vi "GUI_EPS Interface.vi"() -> ()   [LabVIEW 2013]
uses:
  Shared/GUI_Template/GUI_master/tcp_new_data_event.ctl
  Shared/GUI_Template/GUI_master/tcp new data cluster.ctl
panel:
  out "tcp data event":T1
  in  "Refresh Button":bool
  out "statusfloatarrayname.var 1-0::1":string caption="NAME"
  out "statusfloatarrayname.var 1-1::1":string caption="NAME"
  out "statusfloatarray.var 1-0::1":dbl caption="Value" min=0.0 max=0.0
  out "statusfloatarray.var 1-1::1":dbl caption="Value" min=0.0 max=0.0
  out "statusintegerarray.var 1-1::1":i32 caption="Value" min=0 max=0
  out "statusintegerarray.var 1-0::1":i32 caption="Value" min=0 max=10000
  out "statusintegerarrayname.var 1-0::1":string caption="NAME"
  out "statusintegerarrayname.var 1-1::1":string caption="NAME"
  out "statusboolarrayname1.var 1-1::1":string caption="NAME"
  out "statusboolarrayname1.var 1-0::1":string caption="NAME"
  out "statusboolarray1.var 1-1::1":enum16{"off", "on"}(ring) caption="Value"
  out "statusboolarray1.var 1-0::1":enum16{"off", "on"}(ring) caption="Value"
  out "name.var 1-0::1":string caption="NAME"
  in  "variable.var 1-0::1":enum16{"off", "on"}(ring) caption="Toggle"
  in  "insert tag":bool=TRUE
  in  "stop":bool
  in  "GUIdevice 1":string="71146 EPS Interface"
  # "BOOL1"
  # "INTEGER"
  # "FLOAT"
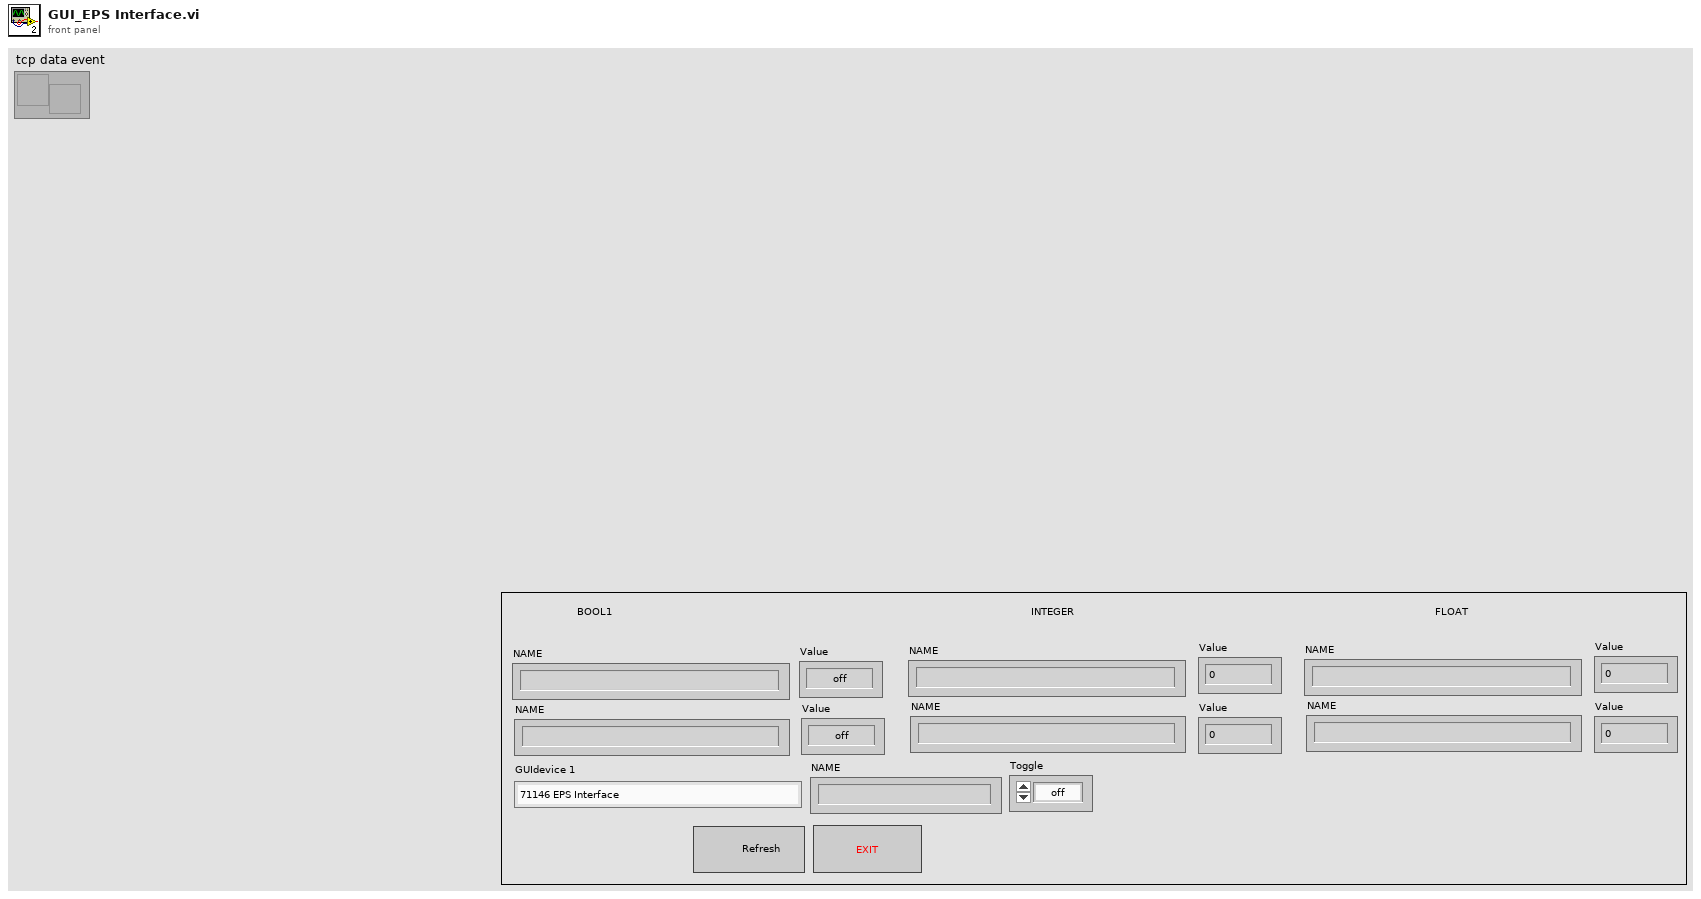
[diagram p1: front panel]
types:
  T1 = typedef "tcp_new_data_event.ctl" = refnum<user-event>
  T2 = enum32{"invalid app kind", "Development System", "Run Time System", "Student Edition", "Embedded LabVIEW", "Evaluation", "Custom"}
  T3 = typedef "tcp new data cluster.ctl" = cluster{"EventEnum":enum16{"new data", "connection status update"}, "Device name":string}
  T4 = enum32{"Invalid", "Standard", "Closed", "Hidden", "Minimized", "Maximized"}
  T5 = cluster{"Core":cluster{"Current VI Reference":refnum<vi>, "Close Panel on Exit?":bool}, "Your Boolean data":bool, "Your string data":string, "SuperGUI":cluster{"STOP queue":refnum<queue>, "SuperGUI ref":refnum<vi>}}
  T6 = cluster{"STOP queue":refnum<queue>, "SuperGUI ref":refnum<vi>}
  T7 = cluster{"Current VI Reference":refnum<vi>, "Close Panel on Exit?":bool}
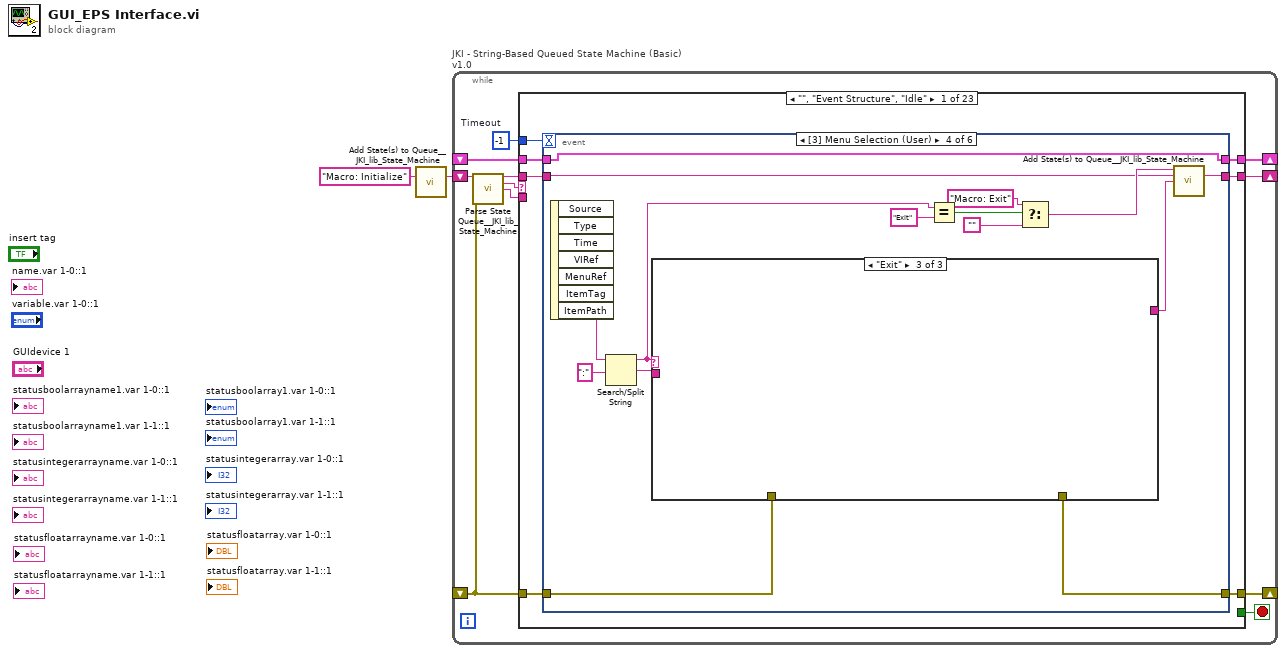
[diagram p0: block diagram]
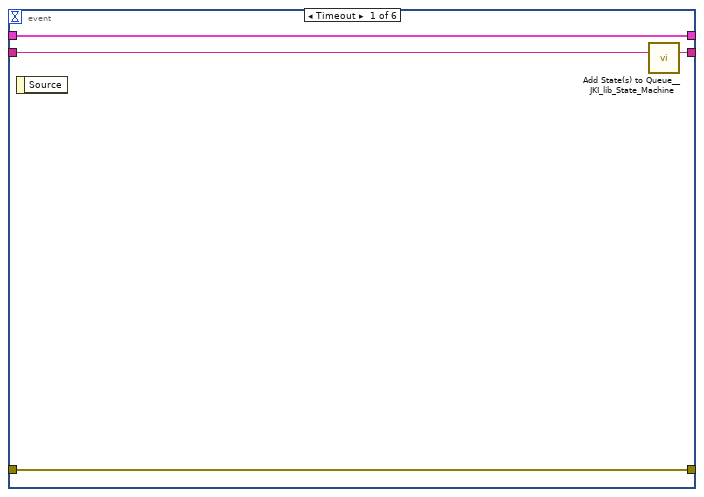
[diagram p2: hidden frame]
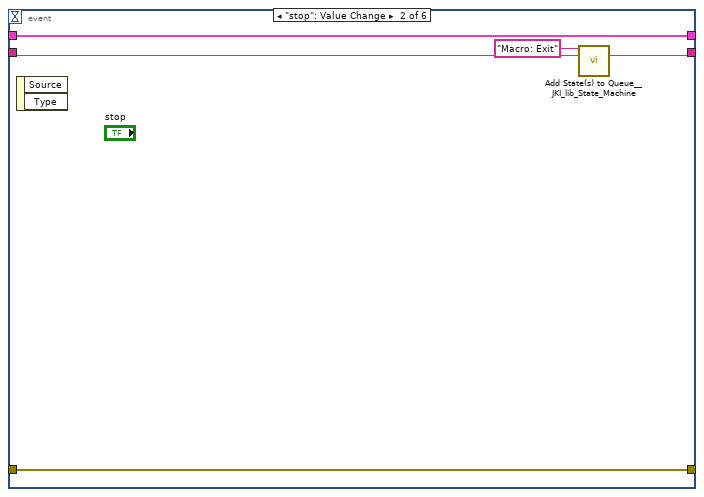
[diagram p3: hidden frame]
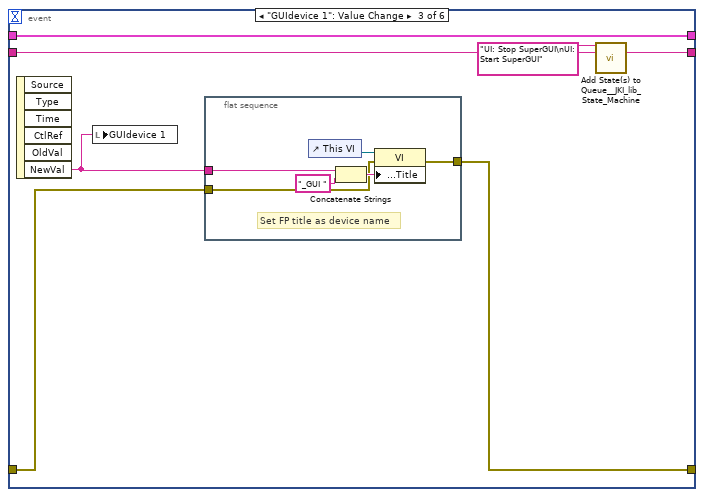
[diagram p4: hidden frame]
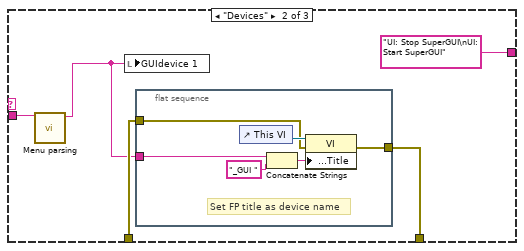
[diagram p6: hidden frame]
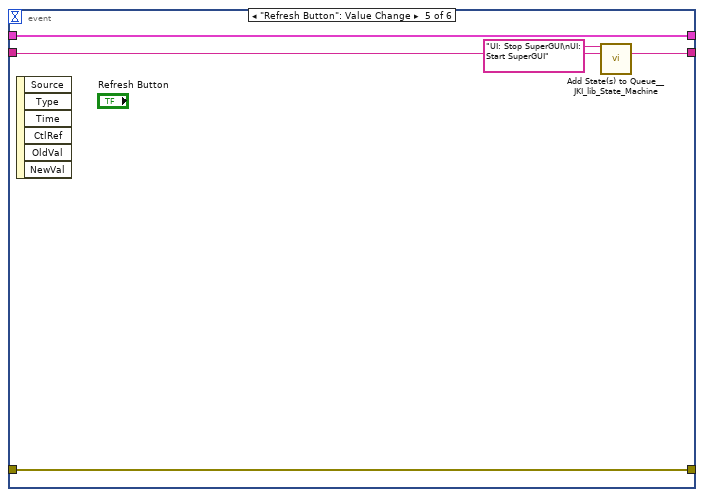
[diagram p7: hidden frame]
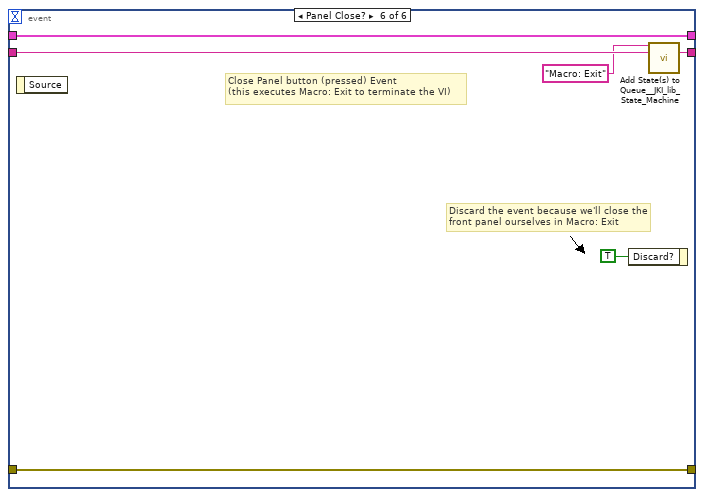
[diagram p8: hidden frame]
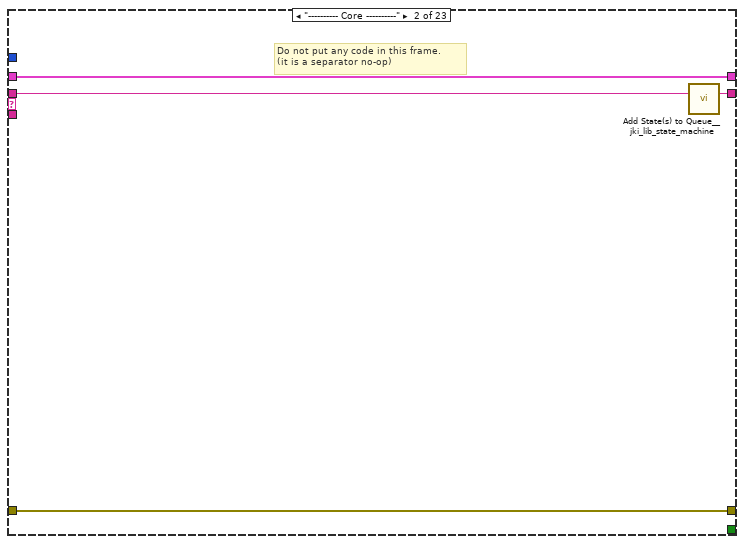
[diagram p9: hidden frame]
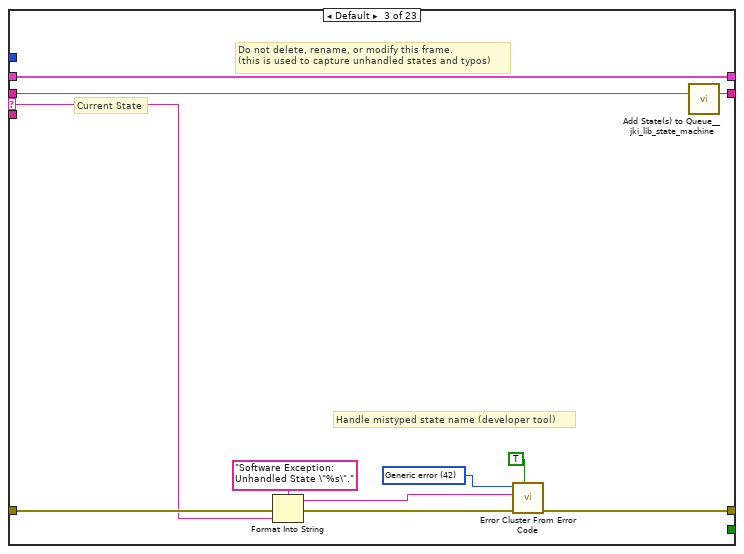
[diagram p10: hidden frame]
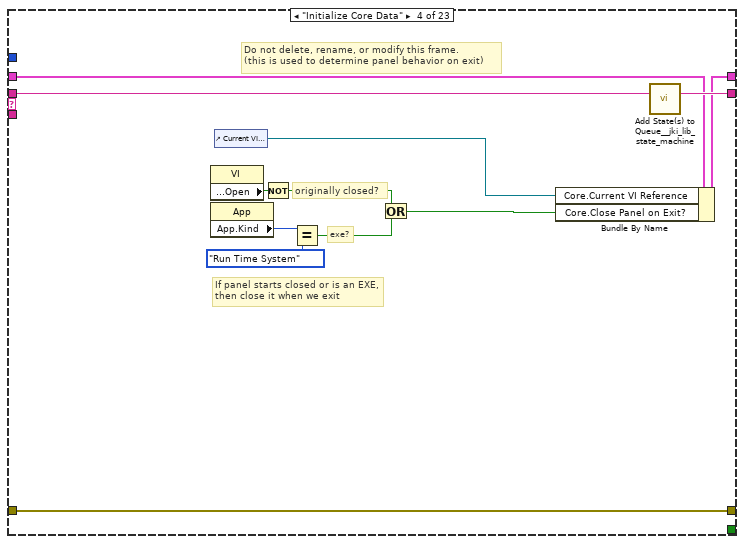
[diagram p11: hidden frame]
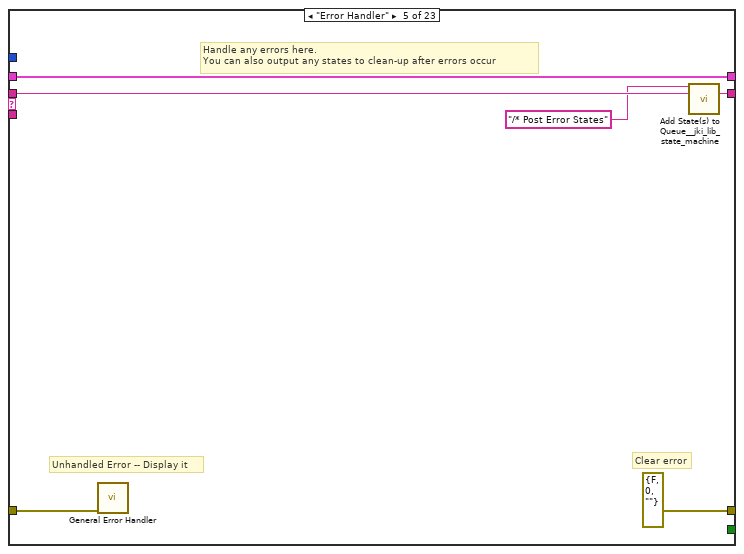
[diagram p12: hidden frame]
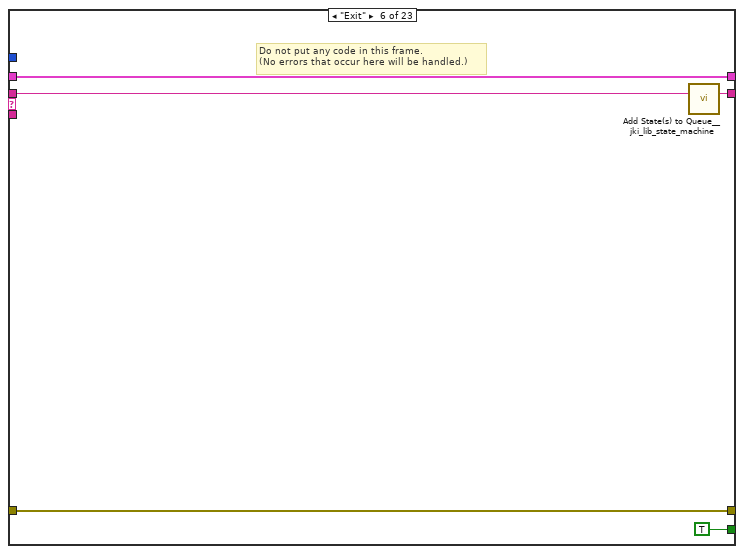
[diagram p13: hidden frame]
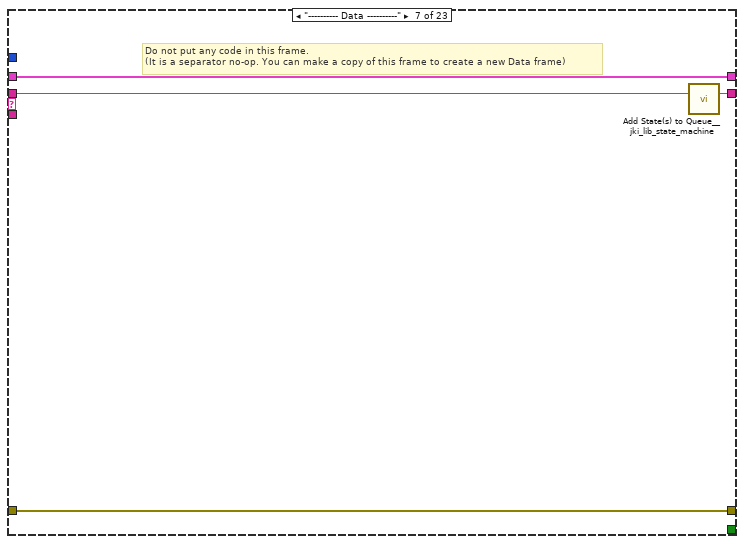
[diagram p14: hidden frame]
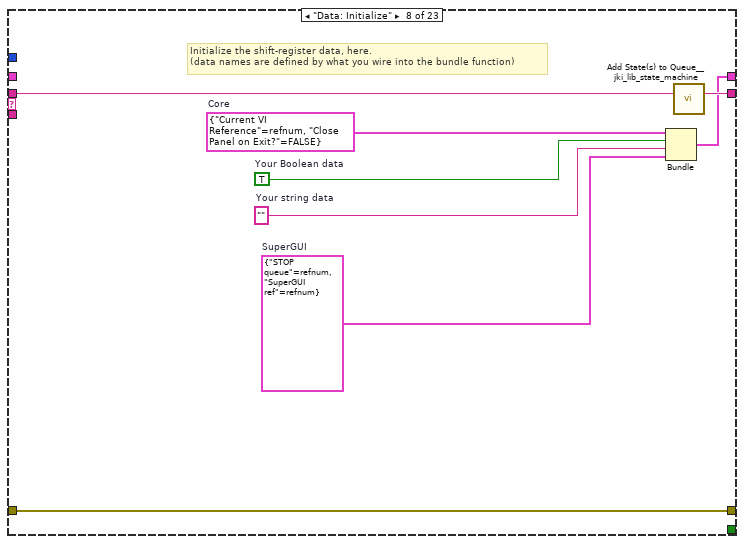
[diagram p15: hidden frame]
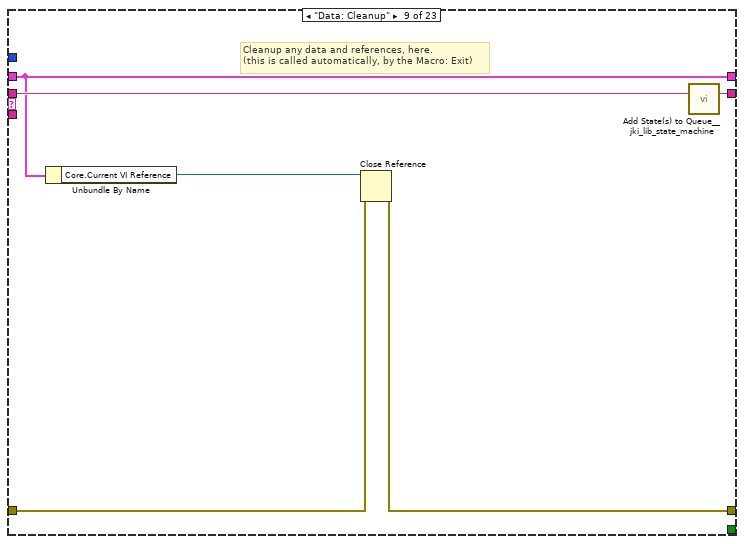
[diagram p16: hidden frame]
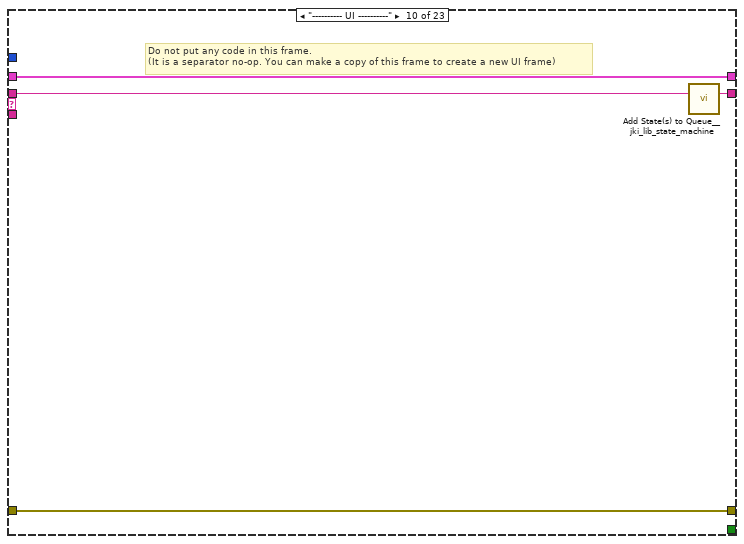
[diagram p17: hidden frame]
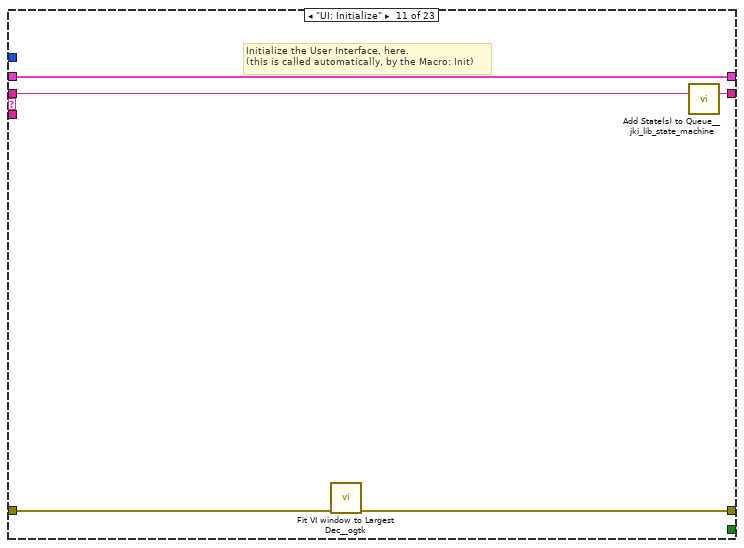
[diagram p18: hidden frame]
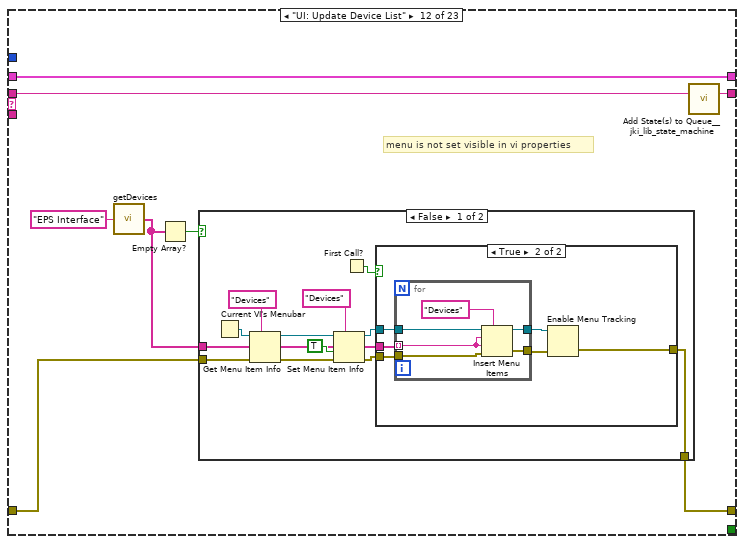
[diagram p19: hidden frame]
diagram:
  n1 = call <vilib>:"Add State(s) to Queue__JKI_lib_State_Machine.vi"("State(s) in (\"\")"="Macro: Initialize") -> ("States Out"=w2:string)  [unwired: 14 in]
  n2 = while "JKI - String-Based Queued State Machine (Basic) v1.0" {
    shift-right: [w6] -> _
    shift-left: _ -> [w5]
    shift-right: [w9] -> _
    shift-left: _ -> [w3]
    shift-right: [w8] -> _
    shift-left: w2 -> [w10]
    stop <- w7 stop-if-true
    w4 = -1  # Timeout
    n3 = call <vilib>:"Parse State Queue__JKI_lib_State_Machine.vi"("State Queue"=w10, "Error In (no error)"=w3) -> ("Remaining States"=w12:string, "Current State"=w13:string, "Arguments"=w11:string)  [unwired: 11 in]
    n4 = case shown="\"\", \"Event Structure\", \"Idle\"" w13 {
      selector: w13 -> [_ _ w86 _ _ _ _ _ _ _ _ _ _ _ _ _ _ _ _ _ _ _ _]
      tunnel: w12 -> [w20 w85 w90 w108 w114 w119 w123 w131 w137 w141 w146 w154 w186 w220 w228 w234 w245 w271 w276 w286 w290 w294 w298]
      tunnel: w11 -> [_ _ _ _ _ _ _ _ _ _ _ _ _ _ _ w229 w239 _ _ _ _ _ _]
      tunnel: w5 -> [w18 w82 w88 w99 w111 w117 w120 _ w132 w138 w144 w152 w184 w211 w223 w232 w241 w268 w273 w283 w287 w291 w295]
      tunnel: [w17 w83 w92 w105 errorcluster {"status"=FALSE, "code"=0, "source"=""} ("error out") w116 w121 w128 w133 w139 w142 w150 w181 w204 w221 w230 w242 w269 w274 w284 w288 w292 w296] -> w9
      tunnel: w3 -> [w16 w83 w91 w105 w110 w116 w121 w128 w134 w139 w143 w151 w182 w205 w222 w231 w243 w269 w274 w284 w288 w292 w296]
      tunnel: [w19 w84 w89 w107 w113 w118 w122 w130 w136 w140 w145 w153 w185 w219 w227 w233 w244 w270 w275 w285 w289 w293 w297] -> w8
      tunnel: [_ _ _ _ _ TRUE _ _ _ _ _ _ _ _ _ _ _ _ _ _ _ _ _] -> w7
      tunnel: [w15 w82 w88 w106 w111 w117 w120 w129 w132 w138 w144 w152 w184 w210 w223 w232 w241 w268 w273 w283 w287 w291 w295] -> w6
      tunnel: w4 -> [w14 _ _ _ _ _ _ _ _ _ _ _ _ _ _ _ _ _ _ _ _ _ _]
      frame "", "Event Structure", "Idle" {
        n5 = event shown="[3] Menu Selection (User)" {
          selector: _ -> [_ _ _ _ _ _]
          dyn-events: _ -> [_ _ _ _ _ _]
          timeout: w14 -> [_ _ _ _ _ _]
          tunnel: w20 -> [w24 w27 w33 w51 w73 w81]
          tunnel: [w23 w26 w32 w50 w72 w80] -> w19
          tunnel: w18 -> [w21 w29 w36 w57 w75 w78]
          tunnel: [w22 w28 w34 w44 w74 w79] -> w17
          tunnel: w16 -> [w22 w28 w35 w45 w74 w79]
          tunnel: [w21 w29 w36 w57 w75 w78] -> w15
          event Timeout {
            n6 = event-data() -> ()  [unwired: 1 in, 1 out]
            n7 = call <vilib>:"Add State(s) to Queue__JKI_lib_State_Machine.vi"("State(s) in (\"\")"=w24) -> ("States Out"=w23:string)  [unwired: 14 in]
          }
          event "stop": Value Change {
            n8 = event-data() -> ()  [unwired: 1 in, 2 out]
            n9 = call <vilib>:"Add State(s) to Queue__JKI_lib_State_Machine.vi"("State(s) in Front (\"\")"="Macro: Exit", "State(s) in (\"\")"=w27) -> ("States Out"=w26:string)  [unwired: 13 in]
          }
          event "GUIdevice 1": Value Change {
            n10 = event-data() -> ("NewVal"=w30:string)  [unwired: 1 in, 5 out]
            n11 = local write "GUIdevice 1"(w30) -> ()
            n12 = flat-sequence {
              tunnel: [w39] -> w34
              tunnel: w35 -> [w38]
              tunnel: w30 -> [w37]
              frame #0 {
                # "Set FP title as device name"
                n13 = control-ref of="This VI"() -> (w42:refnum<vi>)
                n14 = Concatenate Strings(w37, "_GUI ") -> (w41:string)
                n15 = property class="VI"(reference=w42, error in=w38, "Front Panel.Title"=w41) -> (error out=w39:errorcluster)  [unwired: 1 out]
              }
            }
            n16 = call <vilib>:"Add State(s) to Queue__JKI_lib_State_Machine.vi"("State(s) in Front (\"\")"="UI: Stop SuperGUI\nUI: Start SuperGUI", "State(s) in (\"\")"=w33) -> ("States Out"=w32:string)  [unwired: 13 in]
          }
          event Menu Selection (User) {
            n17 = event-data() -> ("ItemPath"=w47:string)  [unwired: 1 in, 6 out]
            n18 = Search/Split String(string=w47, search string/char (-)=":") -> (substring before match=w43:string, match + rest of string=w46:string)  [unwired: 1 in, 1 out]
            n19 = case shown="\"Exit\"" w43 {
              tunnel: w46 -> [_ w63 _]
              tunnel: w45 -> [w58 w62 w70]
              tunnel: [w58 w61 w70] -> w44
              tunnel: [_ "UI: Stop SuperGUI\nUI: Start SuperGUI" _] -> w49
              frame "", Default {
              }
              frame "Devices" {
                n20 = call "Menu parsing.vi"("ItemPath"=w63) -> ("ItemPath"=w59:string)  [unwired: 9 in, 1 out]
                n21 = local write "GUIdevice 1"(w59) -> ()
                n22 = flat-sequence {
                  tunnel: [w66] -> w61
                  tunnel: w62 -> [w65]
                  tunnel: w59 -> [w64]
                  frame #0 {
                    # "Set FP title as device name"
                    n23 = control-ref of="This VI"() -> (w69:refnum<vi>)
                    n24 = Concatenate Strings(w64, "_GUI ") -> (w68:string)
                    n25 = property class="VI"(reference=w69, error in=w65, "Front Panel.Title"=w68) -> (error out=w66:errorcluster)  [unwired: 1 out]
                  }
                }
              }
              frame "Exit" {
              }
            }
            n26 = Equal?(x=w43, y="Exit") -> (x = y?=w55:bool)
            n27 = Select(t="Macro: Exit", s=w55, f="") -> (s? t:f=w52:string)
            n28 = call <vilib>:"Add State(s) to Queue__JKI_lib_State_Machine.vi"("State(s) in Front (\"\")"=w52, "State(s) in (\"\")"=w51, "State(s) at Back (\"\")"=w49) -> ("States Out"=w50:string)  [unwired: 12 in]
          }
          event "Refresh Button": Value Change {
            n29 = event-data() -> ()  [unwired: 1 in, 6 out]
            n30 = call <vilib>:"Add State(s) to Queue__JKI_lib_State_Machine.vi"("State(s) in Front (\"\")"="UI: Stop SuperGUI\nUI: Start SuperGUI", "State(s) in (\"\")"=w73) -> ("States Out"=w72:string)  [unwired: 13 in]
          }
          event Panel Close? {
            # "Discard the event because we'll close the front panel ourselves in Macro: Exit"
            # "Close Panel button (pressed) Event\n(this executes Macro: Exit to terminate the VI)"
            n31 = event-data() -> ()  [unwired: 1 in, 1 out]
            n32 = event-data("Discard?"=TRUE) -> ()  [unwired: 1 in, 1 out]
            n33 = call <vilib>:"Add State(s) to Queue__JKI_lib_State_Machine.vi"("State(s) in Front (\"\")"="Macro: Exit", "State(s) in (\"\")"=w81) -> ("States Out"=w80:string)  [unwired: 13 in]
          }
        }
      }
      frame "---------- Core ----------" {
        # "Do not put any code in this frame.\n(it is a separator no-op)"
        n34 = call <vilib>:"Add State(s) to Queue__jki_lib_state_machine.vi"("State(s) in (\"\")"=w85) -> ("States Out"=w84:string)  [unwired: 14 in]
      }
      frame Default {
        w95 = 42 items=["No error", "Argument error", "Memory is full", "Out of zone", "End of file", "File already open", "Generic file I/O error", "File not found", "File permission error", "Disk is full", "Duplicate path", "Too many files open", "System feature not enabled", "Resource file not found", "Cannot add resource", "Resource not found", "Image not found", "Image memory error", "Pen does not exist", "Config type invalid", "Config token not found", "Config parse error", "Config memory error", "Bad external code format", "Bad external code offset", "External code not present", "Null window", "Destroy window error", "Null menu", "Print aborted", "Bad print record", "Print driver error", "Windows error during printing", "Memory error during printing", "Print dialog error", "Generic print error", "Invalid device refnum", "Device not found", "Device parameter error", "Device unit error", "Cannot open device", "Device call aborted", "Generic error", "Cancelled by user", "Object ID too low", "Object ID too high", "Object not in heap", "Unknown heap", "Unknown object (invalid DefProc)", "Unknown object (DefProc not in table)", "Message out of range", "Invalid (null) method", "Unknown message", "Manager call not supported", "Bad address", "Network operation in progress", "Network operation timed out", "Connection is busy", "Network attribute not supported", "Network error", "Address in use", "System out of memory", "Connection aborted", "Connection refused", "Not connected", "Already connected", "Connection closed", "Initialization error (interapplication manager)", "Bad occurrence", "Wait on unbound occurrence handler", "Occurrence queue overflow", "Datalog type conflict", "Unused", "Unrecognized type (interapplication manager)", "Memory corrupt", "Failed to make temporary DLL", "Old CIN version", "Drag socket not found", "Failed to load drop-object", "Failed to register OLE object", "Failed to release OLE object", "Format specifier type mismatch", "Unknown format specifier", "Too few format specifiers", "Too many format specifiers", "Scan failed", "Newer CIN version", "Error converting to variant", "Runtime menu error", "Password tampered", "Variant attribute not found", "Incompatible variant data type", "Event data is not available", "Event Store is not present", "Occurrence is not found", "Event Queue is not created", "Event info is not available", "Refnum passed is NULL", "Error retrieving Class GUID", "Error retrieving CoClass GUID", "Error retrieving TypeLib GUID.", "Bad built application magic bytes.", "Specific driver is different from the specific driver associated with the Logical Name.", "There is no session opened to the class driver.", "Max Error", "MAX - Error with config objects", "MAX - Error loading configuration", "MAX - Group not supported"]
        # "Current State"
        # "Do not delete, rename, or modify this frame.\n(this is used to capture unhandled states and typos)"
        # "Handle mistyped state name (developer tool)"
        n35 = Format Into String(format string="Software Exception: Unhandled State \"%s\"." ("message"), error in=w91, w86) -> (resulting string=w94:string, error out=w93:errorcluster)  [unwired: 1 in]
        n36 = call <vilib>:"Error Cluster From Error Code.vi"("show call chain? (False)"=TRUE, "error in (no error)"=w93, "error message (\"\")"=w94, "error code (0)"=w95) -> ("error out"=w92:errorcluster)  [unwired: 5 in]
        n37 = call <vilib>:"Add State(s) to Queue__jki_lib_state_machine.vi"("State(s) in (\"\")"=w90) -> ("States Out"=w89:string)  [unwired: 14 in]
      }
      frame "Initialize Core Data" {
        # "Do not delete, rename, or modify this frame.\n(this is used to determine panel behavior on exit)"
        # "originally closed?"
        # "exe?"
        # "If panel starts closed or is an EXE, then close it when we exit"
        n38 = property class="VI"() -> ("Front Panel.Open"=w104:bool)  [unwired: 2 in, 2 out]
        n39 = property class="App"() -> ("App.Kind"=w103:T2)  [unwired: 2 in, 2 out]
        n40 = control-ref of="Current VI Reference"() -> (w97:refnum<vi>)
        n41 = Not(x=w104) -> (.not. x?=w101:bool)
        n42 = Equal?(x=w103, y=T2."Run Time System" ("Application:Kind")) -> (x = y?=w100:bool)
        n43 = Or(x=w101, y=w100) -> (x .or. y?=w98:bool)
        n44 = Bundle By Name(cluster=w99, "Core.Current VI Reference"=w97, "Core.Close Panel on Exit?"=w98) -> (w106:T5)
        n45 = call <vilib>:"Add State(s) to Queue__jki_lib_state_machine.vi"("State(s) in (\"\")"=w108) -> ("States Out"=w107:string)  [unwired: 14 in]
      }
      frame "Error Handler" {
        # "Unhandled Error -- Display it"
        # "Handle any errors here.\nYou can also output any states to clean-up after errors occur"
        # "Clear error"
        n46 = call <vilib>:"General Error Handler.vi"("error in (no error)"=w110) -> ()  [unwired: 10 in, 5 out]
        n47 = call <vilib>:"Add State(s) to Queue__jki_lib_state_machine.vi"("State(s) in Front (\"\")"="/* Post Error States", "State(s) in (\"\")"=w114) -> ("States Out"=w113:string)  [unwired: 13 in]
      }
      frame "Exit" {
        # "Do not put any code in this frame.\n(No errors that occur here will be handled.)"
        n48 = call <vilib>:"Add State(s) to Queue__jki_lib_state_machine.vi"("State(s) in (\"\")"=w119) -> ("States Out"=w118:string)  [unwired: 14 in]
      }
      frame "---------- Data ----------" {
        # "Do not put any code in this frame.\n(It is a separator no-op. You can make a copy of this frame to create a new Data frame)"
        n49 = call <vilib>:"Add State(s) to Queue__jki_lib_state_machine.vi"("State(s) in (\"\")"=w123) -> ("States Out"=w122:string)  [unwired: 14 in]
      }
      frame "Data: Initialize" {
        w124 = T6 {"STOP queue"=refnum, "SuperGUI ref"=refnum}  # SuperGUI
        w125 = T7 {"Current VI Reference"=refnum, "Close Panel on Exit?"=FALSE}  # Core
        w127 = TRUE  # Your Boolean data
        w126 = ""  # Your string data
        # "Initialize the shift-register data, here.\n(data names are defined by what you wire into the bundle function)"
        n50 = Bundle("Core"=w125, "Your Boolean data"=w127, "Your string data"=w126, "SuperGUI"=w124) -> (w129:T5)  [unwired: 1 in]
        n51 = call <vilib>:"Add State(s) to Queue__jki_lib_state_machine.vi"("State(s) in (\"\")"=w131) -> ("States Out"=w130:string)  [unwired: 14 in]
      }
      frame "Data: Cleanup" {
        # "Cleanup any data and references, here.\n(this is called automatically, by the Macro: Exit)"
        n52 = Unbundle By Name(w132) -> ("Core.Current VI Reference"=w135:refnum<vi>)
        n53 = Close Reference(reference=w135, error in (no error)=w134) -> (error out=w133:errorcluster)
        n54 = call <vilib>:"Add State(s) to Queue__jki_lib_state_machine.vi"("State(s) in (\"\")"=w137) -> ("States Out"=w136:string)  [unwired: 14 in]
      }
      frame "---------- UI ----------" {
        # "Do not put any code in this frame.\n(It is a separator no-op. You can make a copy of this frame to create a new UI frame)"
        n55 = call <vilib>:"Add State(s) to Queue__jki_lib_state_machine.vi"("State(s) in (\"\")"=w141) -> ("States Out"=w140:string)  [unwired: 14 in]
      }
      frame "UI: Initialize" {
        # "Initialize the User Interface, here.\n(this is called automatically, by the Macro: Init)"
        n56 = call <userlib>:"Fit VI window to Largest Dec__ogtk.vi"("error in (no error)"=w143) -> ("error out"=w142:errorcluster)  [unwired: 5 in, 1 out]
        n57 = call <vilib>:"Add State(s) to Queue__jki_lib_state_machine.vi"("State(s) in (\"\")"=w146) -> ("States Out"=w145:string)  [unwired: 14 in]
      }
      frame "UI: Update Device List" {
        # "menu is not set visible in vi properties"
        n58 = call "getDevices.vi"("Device Class"="EPS Interface") -> ("All Devices"=w147:string[])
        n59 = Empty Array?(array=w147) -> (empty?=w148:bool)
        n60 = case shown="False" w148 {
          tunnel: w151 -> [w157 w180]
          tunnel: [w156 w180] -> w150
          tunnel: w147 -> [w155 _]
          frame False {
            n61 = Current VI's Menubar() -> (w160:refnum<k9>)
            n62 = Get Menu Item Info(7:"Devices" ("item tag"), 8:w157, 11:w160) -> (0:w166:errorcluster, 3:w162:refnum<k9>)  [unwired: 5 out]
            n63 = Set Menu Item Info(7:"Devices" ("item tag"), 8:w166, 9:TRUE ("enabled"), 11:w162) -> (0:w165:errorcluster, 3:w164:refnum<k9>)  [unwired: 3 in]
            n64 = First Call?() -> (First Call?: T/F=w158:bool)
            n65 = case shown="True" w158 {
              tunnel: w164 -> [_ w172]
              tunnel: w155 -> [_ w171]
              tunnel: w165 -> [w167 w169]
              tunnel: [w167 w168] -> w156
              frame False {
              }
              frame True {
                n66 = for {
                  tunnel: [w179] -> w173
                  tunnel: w171 -> [w177] mode=indexing
                  tunnel: w172 -> [w176]
                  tunnel: [w175] -> w170
                  tunnel: w169 -> [w174]
                  n67 = Insert Menu Items(5:"Devices" ("menu tag"), 6:w174, 7:w177, 8:w177, 9:w176) -> (0:w175:errorcluster, 3:w179:refnum<k9>)  [unwired: 1 in, 1 out]
                }
                n68 = Enable Menu Tracking(2:w170, 4:w173) -> (0:w168:errorcluster)  [unwired: 1 in, 1 out]
              }
            }
          }
          frame True {
          }
        }
        n69 = call <vilib>:"Add State(s) to Queue__jki_lib_state_machine.vi"("State(s) in (\"\")"=w154) -> ("States Out"=w153:string)  [unwired: 14 in]
      }
      frame "UI: Get Device Name" {
        n70 = First Call?() -> (First Call?: T/F=w183:bool)
        n71 = case shown="True" w183 {
          tunnel: w182 -> [w187 w189]
          tunnel: [w187 w188] -> w181
          frame False {
          }
          frame True {
            n72 = disable-structure "Get Device name from control for vi mode\nand command line arg for exe" shown="RUN_TIME_ENGINE==True" {
              disable-tunnel: w189 -> [_ w191]
              disable-tunnel: [_ w190] -> w188
              frame condition #0 (active) {
              }
              frame condition #1 {
                n73 = control-ref of="This Application"() -> (w199:refnum<vi>)
                n74 = property class="App"(reference=w199) -> ("App.Args"=w198:string[])  [unwired: 1 in, 2 out]
                n75 = Index Array(array=w198, index #1=1 ("index")) -> (element #1=w192:string)  [unwired: 2 in, 2 out]
                n76 = Empty String/Path?(string/path=w192) -> (empty?=w196:bool)
                n77 = control-ref of="This VI"() -> (w195:refnum<vi>)
                n78 = case shown="False" w196 {
                  tunnel: w192 -> [w200 _]
                  frame False {
                    n79 = local write "GUIdevice 1"(w200) -> ()
                  }
                  frame True {
                  }
                }
                n80 = Concatenate Strings(w192, "_GUI ") -> (w194:string)
                n81 = property class="VI"(reference=w195, error in=w191, "Front Panel.Title"=w194) -> (error out=w190:errorcluster)  [unwired: 1 out]
              }
            }
          }
        }
        n82 = call <vilib>:"Add State(s) to Queue__jki_lib_state_machine.vi"("State(s) in (\"\")"=w186) -> ("States Out"=w185:string)  [unwired: 14 in]
      }
      frame "UI: Start SuperGUI" {
        # "create stop queue for supergui and its clones"
        # "x100 abort will be dependent on caller VI\nx80 abort will be independent of caller vi, this will abort vi when labview is closed."
        # "Start SuperGUI asynchronous way"
        n83 = vi-ref "GUI_Master_subvi_reentrant_queues.vi"() -> (w203:refnum<vi>)
        n84 = property class="VI"(reference=w203) -> ("Path"=w202:path)  [unwired: 1 in, 2 out]
        n85 = Create User Event(user event datatype=T3 {"EventEnum"=enum."new data", "Device name"="Device name"} ("New Event"), error in=w205) -> (user event=w206:refnum<user-event>, error out=w212:errorcluster)
        "tcp data event" <- w206
        n86 = control-ref of="This Application"() -> (w209:refnum<vi>)
        n87 = control-ref of="This VI"() -> (w208:refnum<vi>)
        n88 = Open VI Reference(type specifier VI Refnum (for type only)=refnum<vi> refnum, vi path=w202, options=256) -> (vi reference=w218:refnum<vi>, error out=w217:errorcluster)  [unwired: 3 in]
        n89 = register-events(w206) -> ()  [unwired: 2 in, 2 out]
        n90 = call "supergui create stop queue.vi"() -> ("STOP Queue out"=w214:refnum<queue>)  [unwired: 11 in]
        n91 = Current VI's Menubar() -> (w207:refnum<k9>)
        n92 = call-by-ref "Start Asynchronous Call"(reference=w218, error in=w217, "STOP Queue in"=w214, "This Application"=w209, 8:"error in (no error)"=w212, "tcp data event"=w206, "Caller menu reference"=w207, "Caller VI ref"=w208) -> (reference out=w201:refnum<vi>, error out=w204:errorcluster)  [unwired: 5 in, 1 out]
        n93 = Bundle By Name(cluster=w211, "SuperGUI.SuperGUI ref"=w201, "SuperGUI.STOP queue"=w214) -> (w210:T5)
        n94 = call <vilib>:"Add State(s) to Queue__jki_lib_state_machine.vi"("State(s) in (\"\")"=w220) -> ("States Out"=w219:string)  [unwired: 14 in]
      }
      frame "UI: Stop SuperGUI" {
        # "Stop Supergui Clone and wait until it exit properly"
        n95 = Unbundle By Name(w223) -> ("SuperGUI.SuperGUI ref"=w225:refnum<vi>, "SuperGUI.STOP queue"=w224:refnum<queue>)
        n96 = Release Queue(queue=w224, error in (no error)=w222) -> (error out=w226:errorcluster)  [unwired: 1 in, 2 out]
        n97 = call-by-ref "Wait On Asynchronous Call"(reference=w225, error in=w226) -> ("error out"=w221:errorcluster)  [unwired: 11 in, 2 out]
        n98 = call <vilib>:"Add State(s) to Queue__jki_lib_state_machine.vi"("State(s) in (\"\")"=w228) -> ("States Out"=w227:string)  [unwired: 14 in]
      }
      frame "UI: Cursor Set" {
        # "Argument"
        # "Set and Unset Cursor Busy.\n(Usage: \"UI: Cursor Set >> Busy|Idle\")"
        n99 = case shown="\"Idle\", Default" w229 {
          tunnel: w231 -> [w236 w238]
          tunnel: [w235 w237] -> w230
          frame "Idle", Default {
            n100 = call <vilib>:"Unset Busy.vi"("error in (no error)"=w236) -> ("error out"=w235:errorcluster)  [unwired: 10 in]
          }
          frame "Busy" {
            n101 = call <vilib>:"Set Busy.vi"("error in (no error)"=w238) -> ("error out"=w237:errorcluster)  [unwired: 9 in, 1 out]
          }
        }
        n102 = call <vilib>:"Add State(s) to Queue__jki_lib_state_machine.vi"("State(s) in (\"\")"=w234) -> ("States Out"=w233:string)  [unwired: 14 in]
      }
      frame "UI: Front Panel State" {
        # "Argument"
        # "Set Front Panel Open or Closed\n(Usage: \"UI: Front Panel State >> Open|Close\")"
        n103 = Unbundle By Name(w241) -> ("Core.Current VI Reference"=w240:refnum<vi>)
        n104 = case shown="\"Close\"" w239 {
          tunnel: w243 -> [w249 w262]
          tunnel: [w251 w263] -> w242
          tunnel: w240 -> [w250 w260]
          frame "Open", Default {
            n105 = property class="VI"(reference=w250, error in=w249) -> (reference out=w247:refnum<vi>, error out=w248:errorcluster, "Front Panel.Open"=w246:bool)
            n106 = case shown="False" w246 {
              tunnel: [w254 w257] -> w251
              tunnel: w248 -> [w253 w257]
              tunnel: w247 -> [w252 _]
              frame False {
                n107 = invoke class="VI" method="FP.Open"(reference=w252, error in=w253, "Activate"=TRUE, "State"=T4."Standard") -> (error out=w254:errorcluster)  [unwired: 1 in, 4 out]
              }
              frame True {
              }
            }
          }
          frame "Close" {
            n108 = property class="VI"(reference=w260, error in=w262) -> (reference out=w259:refnum<vi>, error out=w261:errorcluster, "Front Panel.Open"=w258:bool)
            n109 = case shown="True" w258 {
              tunnel: [w264 w267] -> w263
              tunnel: w261 -> [w264 w266]
              tunnel: w259 -> [_ w265]
              frame False {
              }
              frame True {
                n110 = invoke class="VI" method="FP.Close"(reference=w265, error in=w266) -> (error out=w267:errorcluster)  [unwired: 1 in, 2 out]
              }
            }
          }
        }
        n111 = call <vilib>:"Add State(s) to Queue__jki_lib_state_machine.vi"("State(s) in (\"\")"=w245) -> ("States Out"=w244:string)  [unwired: 14 in]
      }
      frame "---------- Macro ----------" {
        # "Do not put any code in this frame.\n(It is a separator no-op. You can make a copy of this frame to create a new Macro frame)"
        n112 = call <vilib>:"Add State(s) to Queue__jki_lib_state_machine.vi"("State(s) in (\"\")"=w271) -> ("States Out"=w270:string)  [unwired: 14 in]
      }
      frame "Macro: Initialize" {
        # "Initialization Macro\n(This is called once, when the VI starts)"
        n113 = call <vilib>:"Add State(s) to Queue__jki_lib_state_machine.vi"("State(s) in Front (\"\")"="Data: Initialize\nInitialize Core Data\nUI: Initialize\nUI: Update Device List\nUI: Get Device Name\nUI: Start SuperGUI\nUI: Front Panel State >> Open", "State(s) in (\"\")"=w276) -> ("States Out"=w275:string)  [unwired: 13 in]
      }
      frame "Macro: Exit" {
        # "Exit Macro\n(This is called once, when the VI exits)"
        n114 = Unbundle By Name(w283) -> ("Core.Close Panel on Exit?"=w282:bool)
        n115 = Select(t="UI: Front Panel State >> Close", s=w282, f="") -> (s? t:f=w279:string)
        n116 = call <vilib>:"Add State(s) to Queue__jki_lib_state_machine.vi"("State(s) in (\"\")"=w279, "State(s) at Back (\"\")"="Data: Cleanup\nExit") -> ("States Out"=w277:string)  [unwired: 13 in]
        n117 = call <vilib>:"Add State(s) to Queue__jki_lib_state_machine.vi"("State(s) in Front (\"\")"=w277, "State(s) in (\"\")"=w286) -> ("States Out"=w285:string)  [unwired: 13 in]
      }
      frame "---------- New Category ----------" {
        # "Template Separator\n(You can make a copy of, or modify, this frame)"
        n118 = call <vilib>:"Add State(s) to Queue__jki_lib_state_machine.vi"("State(s) in (\"\")"=w290) -> ("States Out"=w289:string)  [unwired: 14 in]
      }
      frame "New Category: 1" {
        # "Your code here.\n(You can make a copy of, or modify, this frame)"
        n119 = call <vilib>:"Add State(s) to Queue__jki_lib_state_machine.vi"("State(s) in (\"\")"=w294) -> ("States Out"=w293:string)  [unwired: 14 in]
      }
      frame "New Category: 2" {
        # "Your code here.\n(You can make a copy of, or modify, this frame)"
        n120 = call <vilib>:"Add State(s) to Queue__jki_lib_state_machine.vi"("State(s) in (\"\")"=w298) -> ("States Out"=w297:string)  [unwired: 14 in]
      }
    }
  }
